vi "eraseCI2_img.vi"   [LabVIEW 2013]
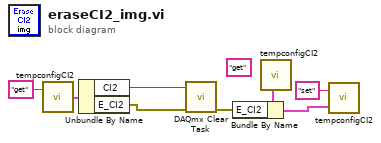
[diagram p0: block diagram]
diagram:
  (unwired) "get" ("command")
  n1 = call "tempconfigCI2.vi"("command"="get") -> ("Temp Config out"=w7:cluster{"CI2":refnum<k21>, "E_CI2":errorcluster})  [unwired: 1 in]
  n2 = Unbundle By Name(w7) -> ("CI2"=w2:refnum<k21>, "E_CI2"=w1:errorcluster)
  n3 = call <vilib>:"DAQmx Clear Task.vi"("task in"=w2, "error in"=w1) -> ("error out"=w4:errorcluster)  [unwired: 13 in]
  n4 = call "tempconfigCI2.vi"() -> ("Temp Config out"=w5:cluster{"CI2":refnum<k21>, "E_CI2":errorcluster})  [unwired: 2 in]
  n5 = Bundle By Name(cluster=w5, "E_CI2"=w4) -> (w3:cluster{"CI2":refnum<k21>, "E_CI2":errorcluster})
  n6 = call "tempconfigCI2.vi"("Temp Config in"=w3, "command"="set") -> ()  [unwired: 1 out]
